vi "Get SSID.vi"() -> (3 "SSID":string)   [LabVIEW 2016, in "Lab Streaming Layer.lvlib"]
uses:
  Lab Streaming Layer.lvlib
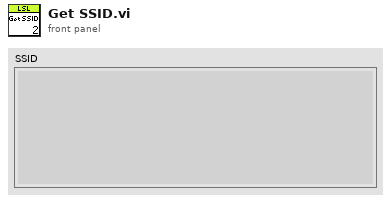
[diagram p1: front panel]
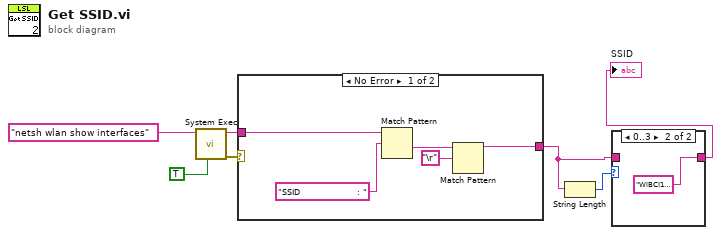
[diagram p0: block diagram]
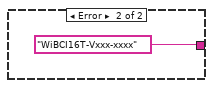
[diagram p3: hidden frame]
diagram:
  n1 = call <vilib>:"System Exec.vi"("run minimized? (F)"=TRUE, "command line"="netsh wlan show interfaces") -> ("error out"=w4:errorcluster, "standard output"=w3:string)  [unwired: 6 in, 2 out]
  n2 = case shown="No Error" w4 {
    tunnel: w3 -> [w12 _]
    tunnel: [w8 "WiBCI16T-Vxxx-xxxx"] -> w6
    frame No Error {
      n3 = Match Pattern(string=w12, regular expression="SSID                   : ") -> (after substring=w10:string)  [unwired: 1 in, 3 out]
      n4 = Match Pattern(string=w10, regular expression="\r") -> (before substring=w8:string)  [unwired: 1 in, 3 out]
    }
    frame Error {
    }
  }
  n5 = String Length(string=w6) -> (length=w5:i32)
  n6 = case shown="0..3" w5 {
    tunnel: w6 -> [w14 _]
    tunnel: [w14 "WiBCI16T-Vxxx-xxxx"] -> w7
    frame 4, Default {
    }
    frame 0..3 {
    }
  }
  "SSID" <- w7
